vi "Parte1_Medicion remota.vi"() -> ()   [LabVIEW 2020]
uses:
  <vilib>/httpClient/LabVIEWHTTPClient.lvlib
panel:
  out "Boolean":bool
  out "Data":string
  out "Hora":string
  out "Accionamiento":dbl
  out "error out":errorcluster
  out "headers":string
  out "body":string
  in  "stop":bool
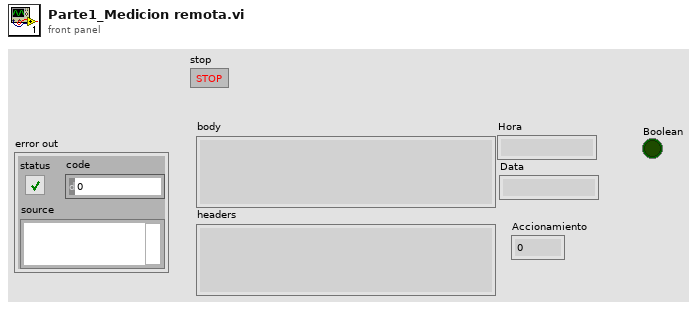
[diagram p1: front panel]
types:
  T1 = cluster{"Accionamiento":dbl, "Data":string, "Hora":string, "Rele":bool}
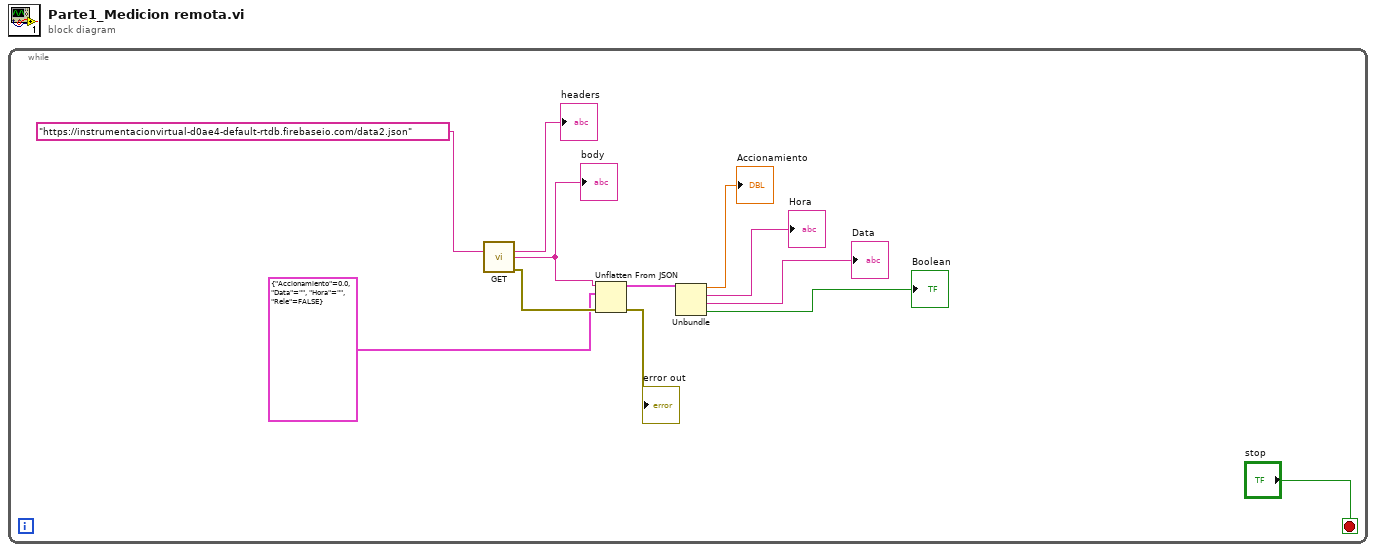
[diagram p0: block diagram]
diagram:
  n1 = while {
    stop <- "stop" stop-if-true
    n2 = call <vilib>:"GET.vi"("url"="https://instrumentacionvirtual-d0ae4-default-rtdb.firebaseio.com/data2.json") -> ("headers"=→"headers":string, "body"=w9:string, "error out"=w8:errorcluster)  [unwired: 11 in, 1 out]
    "body" <- w9
    n3 = Unflatten From JSON(JSON string=w9, type and defaults=T1 {"Accionamiento"=0.0, "Data"="", "Hora"="", "Rele"=FALSE}, error in (no error)=w8) -> (value=w5:T1, error out=→"error out":errorcluster)  [unwired: 4 in]
    n4 = Unbundle "Unbundle"(w5) -> ("Accionamiento"=→"Accionamiento":dbl, "Data"=→"Hora":string, "Hora"=→"Data":string, "Rele"=→"Boolean":bool)
  }
